vi "Get Connection List.vi"(8 "error in (no error)":errorcluster, 11 "PIPXI40 Matrix in":refnum<class "PIPXI40 Matrix.lvclass">) -> (0 "error out":errorcluster, 2 "List":variant, 3 "PIPXI40 Matrix out":refnum<class "PIPXI40 Matrix.lvclass">)   [LabVIEW 2020, in "PIPXI40.lvlib" / "PIPXI40 Matrix.lvclass"]
uses:
  PIPXI40 Matrix.lvclass
  D:/WSGitHub/RTFWK/Realization/PIPXI40 Base/PIPXI40 Base.lvclass
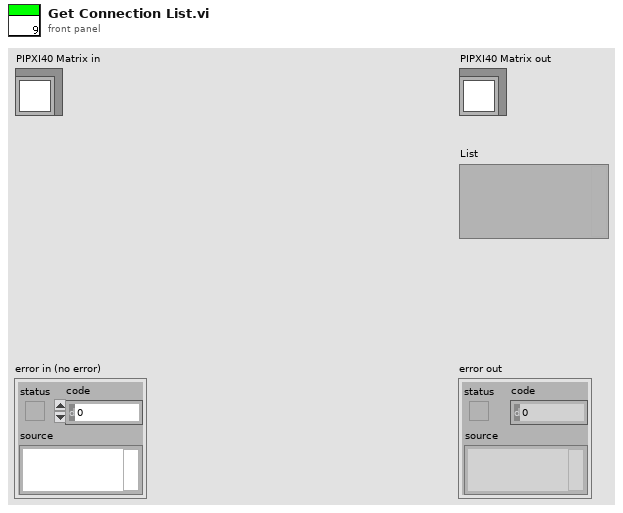
[diagram p1: front panel]
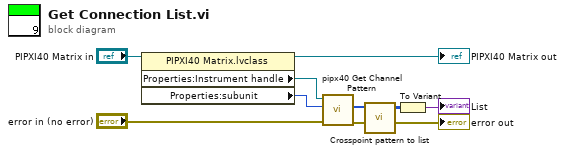
[diagram p0: block diagram]
diagram:
  n1 = property class="PIPXI40 Matrix.lvclass"(reference="PIPXI40 Matrix in") -> (reference out=→"PIPXI40 Matrix out":refnum<class "PIPXI40 Matrix.lvclass">, "Properties:Instrument handle"=w6:refnum<visa-resource-name>, "Properties:subunit"=w1:u32)  [unwired: 1 in, 1 out]
  n2 = call <instrlib>:"pipx40 Get Channel Pattern.vi"("error in (no error)"="error in (no error)", "subunit number"=w1, "instrument handle"=w6) -> ("error out"=→"error out":errorcluster, "pattern"=w4:u32[])  [unwired: 6 in, 1 out]
  n3 = call "Crosspoint pattern to list.vi"("Pattern"=w4) -> ("List"=w2:i32[][])  [unwired: 10 in]
  n4 = To Variant(anything=w2) -> (Variant=→"List":variant)
